vi "Module Init.vi"(8 "error in (no error)":errorcluster, 11 "DAQmxDI in":refnum<class "DAQmxDI.lvclass">) -> (0 "error out":errorcluster, 3 "DAQmxDI out":refnum<class "DAQmxDI.lvclass">)   [LabVIEW 2023, in "VolatusDAQ.lvlib" / "DAQmxDI.lvclass"]
uses:
  DAQmxDI.lvclass
  Volatus/Module/Module.lvclass
  VolatusData/Data Processor Module/Data Processor Module.lvclass
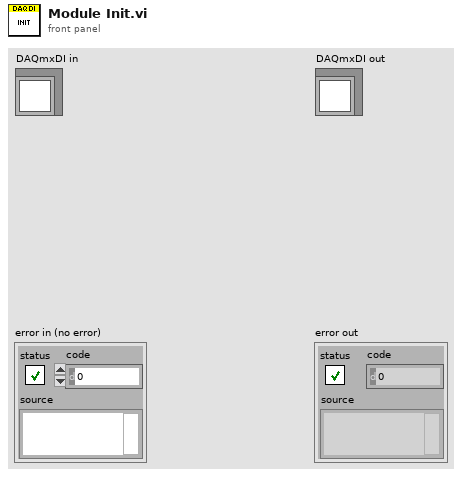
[diagram p1: front panel]
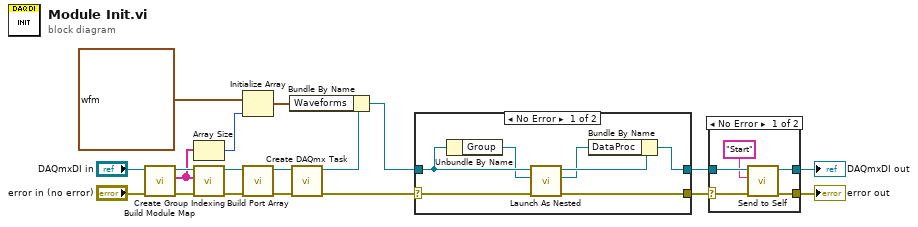
[diagram p0: block diagram]
diagram:
  n1 = call "Build Module Map.vi"("error in (no error)"="error in (no error)", "DAQmxDI in"="DAQmxDI in") -> ("error out"=w14:errorcluster, "Channels"=w5:string[], "DAQmxDI out"=w11:refnum<class "DAQmxDI.lvclass">)  [unwired: 7 in]
  n2 = Array Size(array=w5) -> (size(s)=w4:i32)
  n3 = call "Create Group Indexing.vi"("error in (no error)"=w14, "Channels"=w5, "DAQmxDI in"=w11) -> ("error out"=w12:errorcluster, "DAQmxDI out"=w7:refnum<class "DAQmxDI.lvclass">)  [unwired: 7 in]
  n4 = Initialize Array(waveform(dbl) {"t0"=timestamp(0 s since 1904-01-01), "dt"=1.0, "Y"=[]} ("Waveform"), w4) -> (w1:waveform(dbl)[])
  n5 = call "Build Port Array.vi"("error in (no error)"=w12, "DAQmxDI in"=w7) -> ("error out"=w8:errorcluster, "DAQmxDI out"=w6:refnum<class "DAQmxDI.lvclass">)  [unwired: 8 in]
  n6 = call "Create DAQmx Task.vi"("error in (no error)"=w8, "DAQmxDI in"=w6) -> ("error out"=w10:errorcluster, "DAQmxDI out"=w9:refnum<class "DAQmxDI.lvclass">)  [unwired: 8 in]
  n7 = Bundle By Name(cluster=w9, "Waveforms"=w1) -> (w2:refnum<class "DAQmxDI.lvclass">)
  n8 = case shown="No Error" w10 {
    selector: w10 -> [w26 w27]
    tunnel: w2 -> [w22 w28]
    tunnel: [w23 w27] -> w19
    tunnel: [w24 w28] -> w18
    frame No Error {
      n9 = Unbundle By Name(w22) -> ("Group"=w21:refnum<class "Group DBL.lvclass">)
      n10 = call "Launch As Nested.vi"("error in (no error)"=w26, "Group"=w21, "Parent in"=w22) -> ("error out"=w23:errorcluster, "MessageQ"=w20:refnum<class "MessageQ.lvclass">, "Parent out"=w25:refnum<class "DAQmxDI.lvclass">)  [unwired: 6 in]
      n11 = Bundle By Name(cluster=w25, "DataProc"=w20) -> (w24:refnum<class "DAQmxDI.lvclass">)
    }
    frame Error {
    }
  }
  n12 = case shown="No Error" w19 {
    selector: w19 -> [w33 w35]
    tunnel: [w32 w35] -> w15
    tunnel: w18 -> [w31 w34]
    tunnel: [w30 w34] -> w16
    frame No Error {
      n13 = call "Send to Self.vi"("error in (no error)"=w33, "Message ID"="Start", "Module in"=w31) -> ("error out"=w32:errorcluster, "Module out"=w30:refnum<class "DAQmxDI.lvclass">)  [unwired: 7 in]
    }
    frame Error {
    }
  }
  "error out" <- w15
  "DAQmxDI out" <- w16
